vi "G_PalaDeGrua.vi"() -> ()   [LabVIEW 2020]
panel:
  out "Pala de grua":bool
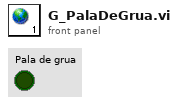
[diagram p1: front panel]
diagram:
